vi "TDTSyn-Get Spikes.vi"(0 "TTankX":refnum<k7>, 1 "TankCode":string, 5 "T1":dbl, 9 "offset":i32, 11 "error in (no error)":errorcluster, 12 "Max Read":i32=1000, 13 "Tetrode":bool) -> (4 "Got 'em all":bool, 8 "Spike times":dbl[][](array[numeric]), 14 "Last Time":dbl, 15 "error out":errorcluster)   [LabVIEW 2020]
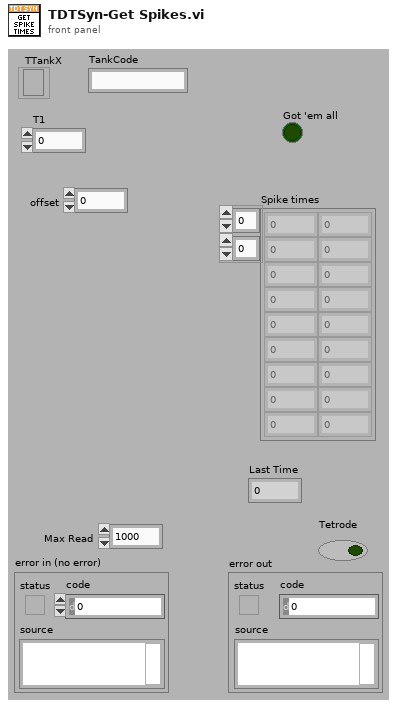
[diagram p1: front panel]
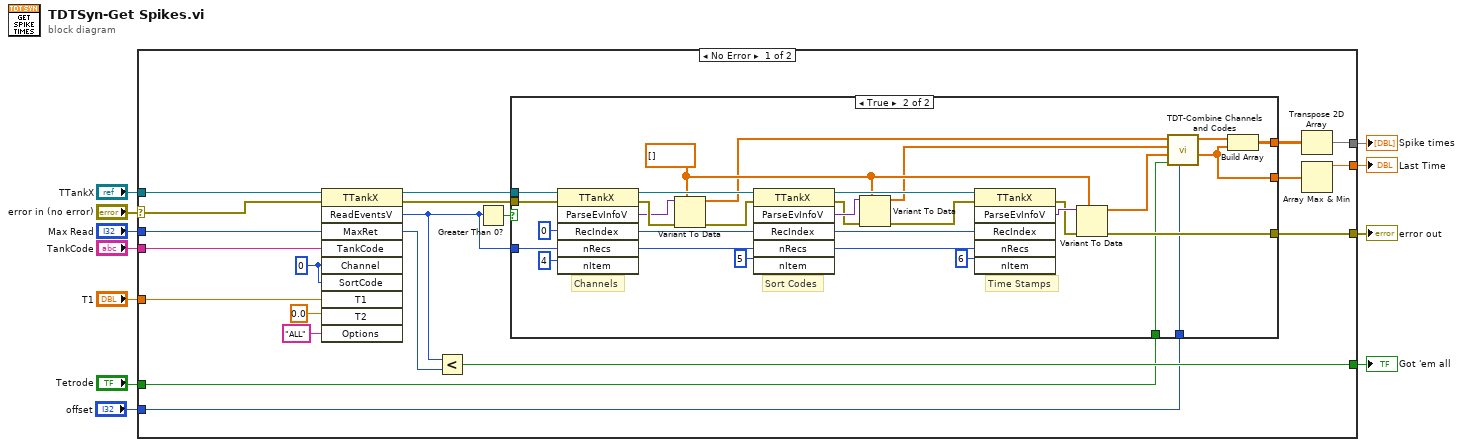
[diagram p0: block diagram]
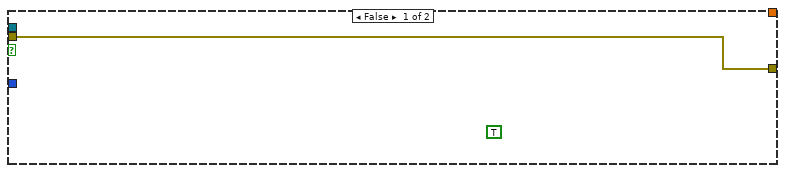
[diagram p2: hidden frame]
diagram:
  n1 = case shown="No Error" "error in (no error)" {
    selector: "error in (no error)" -> [w32 w65]
    tunnel: "Max Read" -> [w31 _]
    tunnel: [w17 w65] -> w9
    tunnel: [w30 _] -> w8
    tunnel: [w19 _] -> w7
    tunnel: [w18 _] -> w6
    tunnel: "Tetrode" -> [w16 _]
    tunnel: "TTankX" -> [w15 _]
    tunnel: "TankCode" -> [w14 _]
    tunnel: "T1" -> [w13 _]
    tunnel: "offset" -> [w12 _]
    frame No Error {
      w26 = 0 ("Channel")
      n2 = invoke class="TTankX" method="ReadEventsV"(reference=w15, error in=w32, "MaxRet"=w31, "TankCode"=w14, "Channel"=w26, "SortCode"=w26, "T1"=w13, "T2"=0.0, "Options"="ALL") -> (reference out=w24:refnum<k7>, error out=w23:errorcluster, "ReadEventsV"=w21:i32, "MaxRet"=w25:i32)  [unwired: 1 in, 6 out]
      n3 = Less?(x=w21, y=w25) -> (x < y?=w18:bool)
      n4 = Greater Than 0?(x=w21) -> (x > 0?=w22:bool)
      n5 = case shown="True" w22 {
        tunnel: w24 -> [_ w64]
        tunnel: w23 -> [w33 w63]
        tunnel: w21 -> [_ w61]
        tunnel: [_ w38] -> w29
        tunnel: [w33 w56] -> w17
        tunnel: [_ w35] -> w20
        tunnel: w16 -> [_ w37]
        tunnel: w12 -> [_ w34]
        frame False {
          (unwired) TRUE
        }
        frame True {
          w43 = dbl[] []
          # "Time Stamps"
          # "Sort Codes"
          # "Channels"
          n6 = invoke class="TTankX" method="ParseEvInfoV"(reference=w64, error in=w63, "RecIndex"=0, "nRecs"=w61, "nItem"=4) -> (reference out=w53:refnum<k7>, error out=w59:errorcluster, "ParseEvInfoV"=w54:variant, "RecIndex"=w51:i32, "nRecs"=w50:i32)  [unwired: 1 in, 1 out]
          n7 = Variant To Data(error in=w59, type=w43, Variant=w54) -> (data=w41:dbl[], error out=w44:errorcluster)
          n8 = invoke class="TTankX" method="ParseEvInfoV"(reference=w53, error in=w44, "RecIndex"=w51, "nRecs"=w50, "nItem"=5) -> (reference out=w52:refnum<k7>, error out=w45:errorcluster, "ParseEvInfoV"=w46:variant, "RecIndex"=w47:i32, "nRecs"=w48:i32)  [unwired: 1 in, 1 out]
          n9 = Variant To Data(error in=w45, type=w43, Variant=w46) -> (data=w40:dbl[], error out=w39:errorcluster)
          n10 = invoke class="TTankX" method="ParseEvInfoV"(reference=w52, error in=w39, "RecIndex"=w47, "nRecs"=w48, "nItem"=6) -> (error out=w55:errorcluster, "ParseEvInfoV"=w57:variant)  [unwired: 1 in, 4 out]
          n11 = Variant To Data(error in=w55, type=w43, Variant=w57) -> (data=w36:dbl[], error out=w56:errorcluster)
          n12 = call "TDT-Combine Channels and Codes.vi"("offset"=w34, "Tetrode"=w37, "Times"=w36, "Sort Codes"=w40, "Channels"=w41) -> ("Times Out"=w35:dbl[], "Impale channel"=w42:dbl[])  [unwired: 5 in]
          n13 = Build Array(w42, w35) -> (w38:dbl[][])
        }
      }
      n14 = Transpose 2D Array(2D array=w29) -> (transposed array=w30:dbl[][])
      n15 = Array Max & Min(array=w20) -> (max value=w19:dbl)  [unwired: 3 out]
    }
    frame Error {
    }
  }
  "Spike times" <- w8
  "error out" <- w9
  "Last Time" <- w7
  "Got 'em all" <- w6
